vi "Read PNG iTXt Chunk.vi"(10 "error in (no error)":errorcluster, 11 "data":u8[](array[numeric])) -> (2 "error out":errorcluster, 3 "String":string)   [LabVIEW 2021, in "Files.lvlib"]
uses:
  Files.lvlib
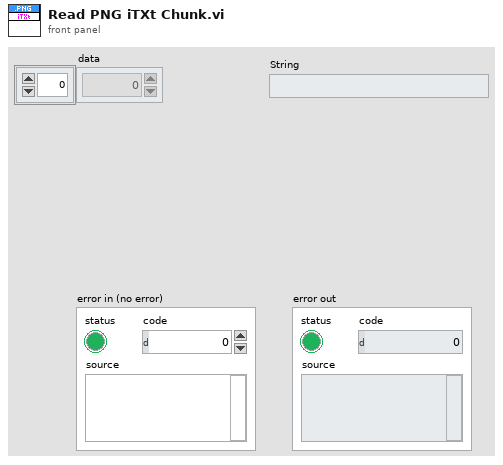
[diagram p1: front panel]
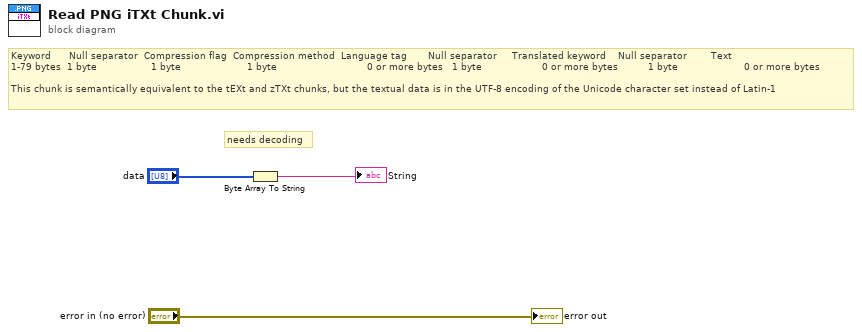
[diagram p0: block diagram]
diagram:
  # "needs decoding"
  # "Keyword      Null separator \tCompression flag \tCompression method \tLanguage tag \t     Null separator \t   Translated keyword   \tNull separator \t      Text\n1-79 bytes \t1 byte \t                1 byte \t                    1 byte \t                            0 or more bytes \t 1 byte \t                  0 or more bytes \t        1 byte \t                    0 or more bytes\n \nThis chunk is semantically equivalent to the tEXt and zTXt chunks, but the textual data is in the UTF-8 encoding of the Unicode character set instead of Latin-1"
  n1 = Byte Array To String(unsigned byte array="data") -> (string=→"String":string)
  "error out" <- "error in (no error)"
